vi "PointsToROI.vi"(6 "Clear Motion Planes":bool, 9 "Old ROIs":T1(array[cluster]), 11 "Points":dbl[][](array[numeric])) -> (3 "ROIs":T1(array[cluster]))   [LabVIEW 2014]
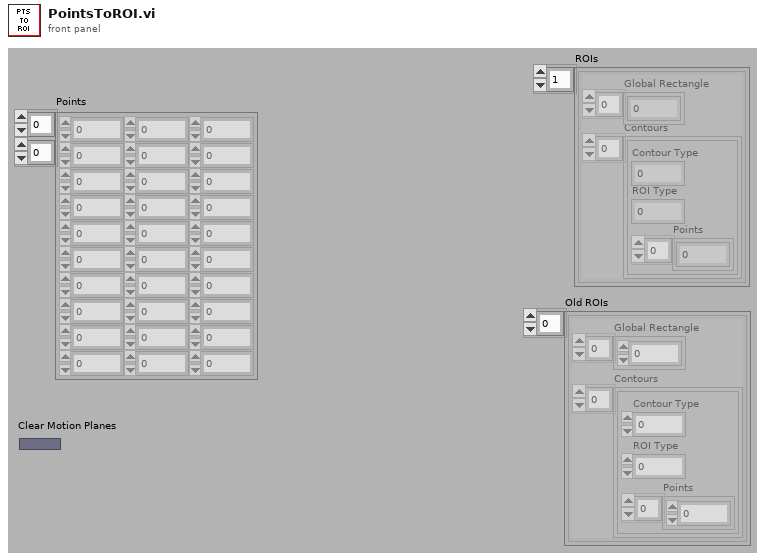
[diagram p1: front panel]
types:
  T1 = cluster{"Global Rectangle":i32[], "Contours":cluster{"Contour Type":u32, "ROI Type":u32, "Points":i32[]}[]}[]
  T2 = cluster{"Global Rectangle":i32[], "Contours":cluster{"Contour Type":u32, "ROI Type":u32, "Points":i32[]}[]}
  T3 = cluster{"Contour Type":u32, "ROI Type":u32, "Points":i32[]}[]
  T4 = cluster{"Contour Type":u32, "ROI Type":i32, "Points":i32[]}
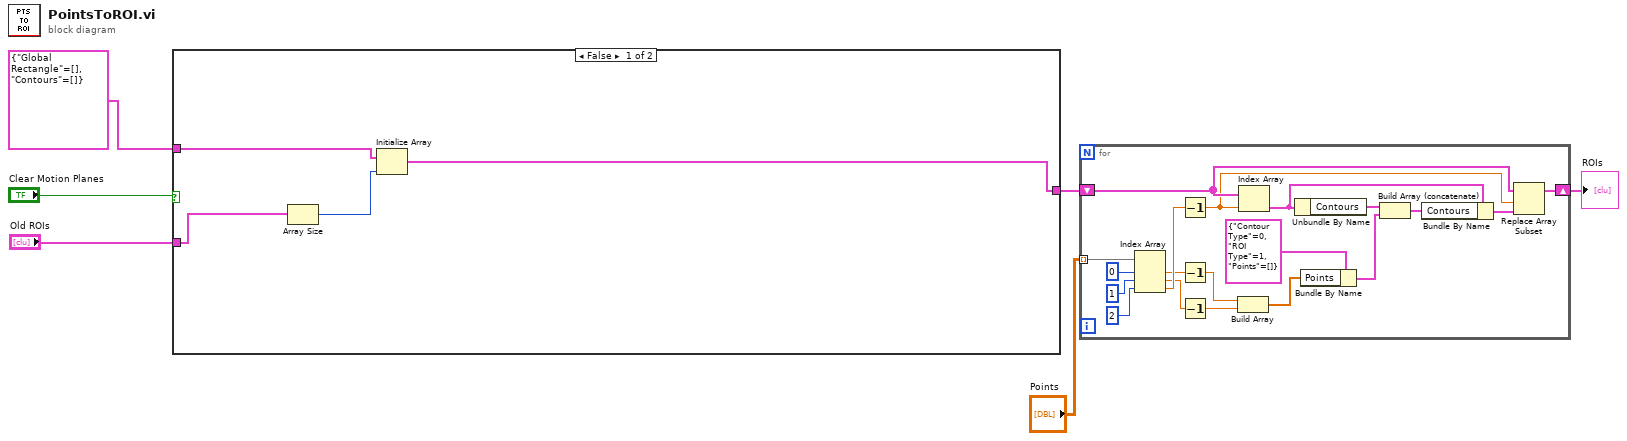
[diagram p0: block diagram]
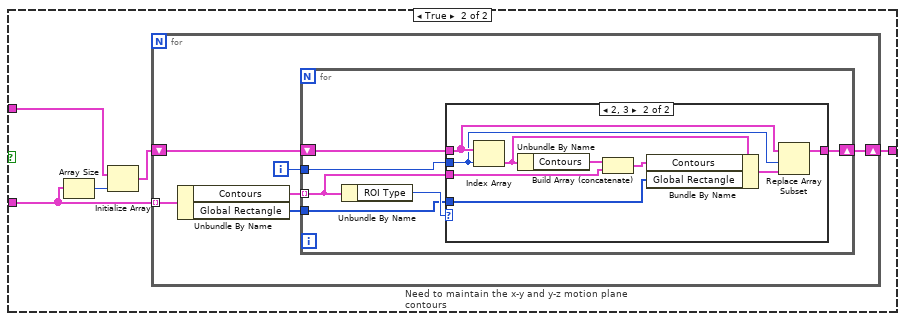
[diagram p2: hidden frame]
diagram:
  n1 = case shown="False" "Clear Motion Planes" {
    tunnel: "Old ROIs" -> [w8 w15]
    tunnel: T2 {"Global Rectangle"=[], "Contours"=[]} ("ROI") -> [w10 w14]
    tunnel: [w9 w11] -> w2
    frame False {
      n2 = Array Size(array=w8) -> (size(s)=w7:i32)
      n3 = Initialize Array(w10, w7) -> (w9:T1)
    }
    frame True {
      n4 = Array Size(array=w15) -> (size(s)=w13:i32)
      n5 = Initialize Array(w14, w13) -> (w12:T1)
      n6 = for "Need to maintain the x-y and y-z motion plane contours" {
        shift-right: [w17] -> w11
        shift-left: w12 -> [w19]
        tunnel: w15 -> [w20] mode=indexing
        i -> [w18]
        n7 = Unbundle By Name(w20) -> ("Contours"=w21:T3, "Global Rectangle"=w16:i32[])
        n8 = for {
          tunnel: w21 -> [w24] mode=indexing
          shift-right: [w23] -> w17
          shift-left: w19 -> [w26]
          tunnel: w18 -> [w25]
          tunnel: w16 -> [w22]
          n9 = Unbundle By Name(w24) -> ("ROI Type"=w27:u32)
          n10 = case shown="2, 3" w27 {
            tunnel: w26 -> [w28 w33]
            tunnel: w25 -> [_ w32]
            tunnel: w24 -> [_ w37]
            tunnel: [w28 w30] -> w23
            tunnel: w22 -> [_ w29]
            frame 0, 1, Default {
            }
            frame 2, 3 {
              n11 = Index Array(array=w33, index=w32) -> (element=w34:T2)
              n12 = Unbundle By Name(w34) -> ("Contours"=w36:T3)
              n13 = Build Array (concatenate)(w36, w37) -> (w35:T3)
              n14 = Bundle By Name(cluster=w34, "Contours"=w35, "Global Rectangle"=w29) -> (w31:T2)
              n15 = Replace Array Subset(array=w33, new element=w31, index=w32) -> (w30:T1)
            }
          }
        }
      }
    }
  }
  n16 = for {
    tunnel: "Points" -> [w56] mode=indexing
    shift-right: [w44] -> w5
    shift-left: w2 -> [w48]
    n17 = Index Array(array=w56, index #1=0 ("index"), index #2=1 ("index"), index #3=2 ("index")) -> (element #1=w39:dbl, element #2=w41:dbl, element #3=w54:dbl)
    n18 = Decrement(x=w54) -> (x-1=w47:dbl)
    n19 = Decrement(x=w39) -> (x-1=w38:dbl)
    n20 = Decrement(x=w41) -> (x-1=w40:dbl)
    n21 = Build Array(w38, w40) -> (w45:dbl[])
    n22 = Index Array(array=w48, index=w47) -> (element=w52:T2)
    n23 = Unbundle By Name(w52) -> ("Contours"=w53:T3)
    n24 = Bundle By Name(cluster=T4 {"Contour Type"=0, "ROI Type"=1, "Points"=[]}, "Points"=w45) -> (w49:T4)
    n25 = Build Array (concatenate)(w53, w49) -> (w51:T3)
    n26 = Bundle By Name(cluster=w52, "Contours"=w51) -> (w46:T2)
    n27 = Replace Array Subset(array=w48, new element=w46, index=w47) -> (w44:T1)
  }
  "ROIs" <- w5
